vi "LINXx - Custom commands.vi"() -> ()   [LabVIEW 2019]
uses:
  <vilib>/MakerHub/LINX/Public/Utilities/Open Serial.vi
  <vilib>/MakerHub/LINX/LMH-LINX.lvlib
  vi.lib/LINXx/LINXx.lvlib
panel:
  in  "run swell":bool
  in  "Swell time [ms]":u16=1000
  out "Waveform Graph":dbl[](graph)
  in  "stop":bool
  out "Loop Rate (Hz)":u32
  in  "Serial Port":refnum<visa-resource-name>="N/A"
  # "Use Adafruit M0 Custom command firmware for this example\n[in Arduino IDE, \nFile>Examples>LINX>Adafruit_Feather_M0_CustomCommand\nand upload sketch]"
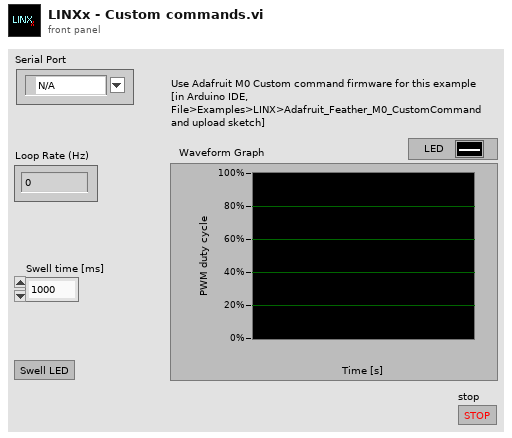
[diagram p1: front panel]
types:
  T1 = typedef "LMH-LINX.lvlib/LINX Ref.ctl" = cluster{"IO":T2, "Interface":T3, "LINX Device Config":T4}
  T2 = typedef "LMH-LINX.lvlib/Platform.ctl" = enum16{"Remote", "Local"}
  T3 = typedef "LMH-LINX.lvlib/Interface.ctl" = enum16{"Serial", "TCP"}
  T4 = typedef "LMH-LINX.lvlib/Device.lvlib/LINX Device Config.ctl" = cluster{"Interface":T3, "COM Port":refnum<visa-resource-name>, "TCP Configuration":T5, "Device Family":u8, "Device ID":u8, "Device Name":string, "TCP Ref":refnum<k5>, "Channels":T6}
  T5 = typedef "LMH-LINX.lvlib/Device.lvlib/TCP Config.ctl" = cluster{"IP Address":string, "Port":u16}
  T6 = typedef "LMH-LINX.lvlib/Channels.ctl" = cluster{"DI":u8[], "DO":u8[], "AI":u8[], "AO":u8[], "PWM":u8[], "QE":u8[], "UART":u8[], "I2C 2":u8[], "SPI":u8[], "CAN":u8[], "Servo":u8[], "AI Ref (V)":dbl, "AI Resolution (Bits)":u8, "AO Ref (V)":dbl, "AO Resolution (Bits)":u8}
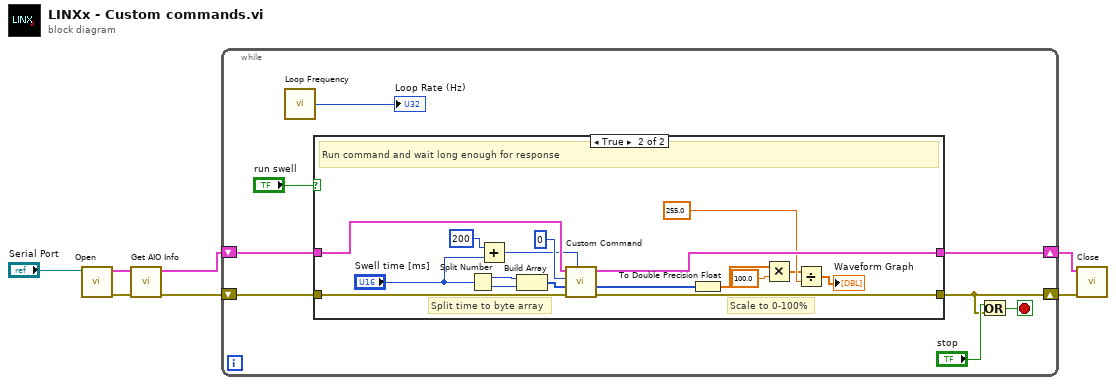
[diagram p0: block diagram]
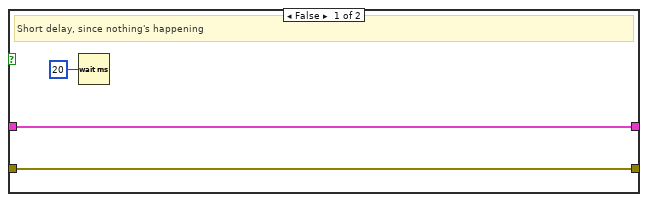
[diagram p2: hidden frame]
diagram:
  n1 = call-poly <vilib>:"Open.vi"("Serial Port"="Serial Port") -> ("Error Out"=w6:errorcluster, "LINX Resource"=w5:T1)  [unwired: 8 in, 1 out]
  n2 = call "Get AIO Info.vi"("Error In"=w6, "LINX Resource"=w5) -> ("Error Out"=w3:errorcluster, "LINX resource"=w4:T1)  [unwired: 6 in, 2 out]
  n3 = while {
    shift-right: [w9] -> w1
    shift-left: w4 -> [w12]
    shift-right: [w10] -> w2
    shift-left: w3 -> [w11]
    stop <- w14 stop-if-true
    n4 = call <vilib>:"Loop Frequency.vi"() -> ("Loop Rate (Hz)"=→"Loop Rate (Hz)":u32)
    n5 = case shown="True" "run swell" {
      tunnel: w12 -> [w16 w35]
      tunnel: w11 -> [w17 w34]
      tunnel: [w17 w33] -> w10
      tunnel: [w16 w32] -> w9
      frame False {
        # "Short delay, since nothing's happening"
        n6 = Wait (ms)(milliseconds to wait=u32 20) -> ()  [unwired: 1 out]
      }
      frame True {
        # "Scale to 0-100%"
        # "Split time to byte array"
        # "Run command and wait long enough for response"
        n7 = Split Number(x="Swell time [ms]") -> (hi(x)=w31:u8, lo(x)=w30:u8)
        n8 = Add(x=u16 200, y="Swell time [ms]") -> (x+y=w25:u16)
        n9 = Build Array(w31, w30) -> (w29:u8[])
        n10 = call <vilib>:"Custom Command.vi"("Timeout (100 ms)"=w25, "Error In"=w34, "Data"=w29, "Custom Command Number"=u16 0, "LINX Resource"=w35) -> ("Error Out"=w33:errorcluster, "Response"=w23:u8[], "LINX Resource"=w32:T1)  [unwired: 3 in, 1 out]
        n11 = To Double Precision Float(number=w23) -> (double precision float=w22:dbl[])
        n12 = Multiply(x=w22, y=100.0 ("Numeric Control")) -> (x*y=w20:dbl[])
        n13 = Divide(x=w20, y=255.0 ("Numeric Control")) -> (x/y=→"Waveform Graph":dbl[])
      }
    }
    n14 = Or(x="stop", y=w10) -> (x .or. y?=w14:bool)
  }
  n15 = call <vilib>:"Close.vi"("Error In"=w2, "LINX Resource"=w1) -> ()  [unwired: 9 in, 1 out]
